vi "Last Ack Event.vi"(10 "Event jettl":refnum<class "Event.lvclass">, 11 "Hello World Queue in":refnum<class "Hello World Queue.lvclass">) -> (3 "Hello World Queue out":refnum<class "Hello World Queue.lvclass">)   [LabVIEW 2021, in "Hello World Queue.lvlib" / "Hello World Queue.lvclass"]
uses:
  Hello World Queue.lvclass
  jettl/Event/Event.lvclass
  Hello World Queue.lvclass/Hello World Queue.ctl
  jettl/Queue/Queue.lvclass
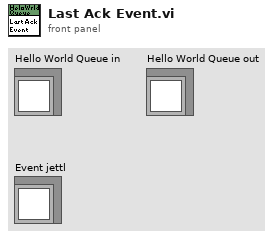
[diagram p1: front panel]
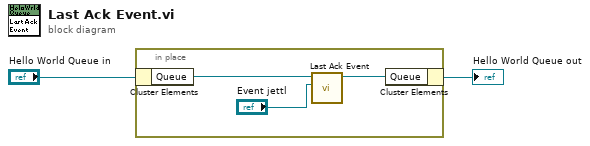
[diagram p0: block diagram]
diagram:
  n1 = in-place {
    n2 = in-place-cluster #1("Hello World Queue in") -> ("Queue"=w5:refnum<class "Queue.lvclass">)
    n3 = call-dynamic "Last Ack Event.vi"("Event"="Event jettl", "Last Ack Event in"=w5) -> ("Last Ack Event out"=w4:refnum<class "Queue.lvclass">)  [unwired: 9 in]
    n4 = in-place-cluster #1("Queue"=w4) -> (→"Hello World Queue out":refnum<class "Hello World Queue.lvclass">)
  }
